vi "addion labview.vi"() -> ()   [LabVIEW 2020]
panel:
  out "x = y?":bool
  in  "x":dbl
  in  "y":dbl
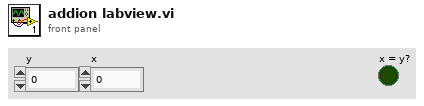
[diagram p1: front panel]
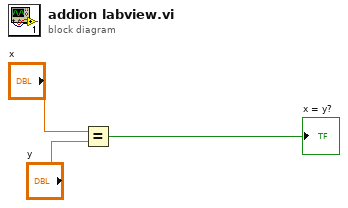
[diagram p0: block diagram]
diagram:
  n1 = Equal?(x="x", y="y") -> (x = y?=→"x = y?":bool)
